vi "SaveGeneralConfigData.vi"(10 "Configurations":T2, 11 "Refnum in":T1) -> (3 "Refnum out":T1)   [LabVIEW 2014]
uses:
  <vilib>/Utility/config.llb/Config Data RefNum.ctl
  <vilib>/Utility/config.llb/Write Key (I32).vi
  <vilib>/Utility/config.llb/NI_LVConfig.lvlib
panel:
  out "error out 3":errorcluster
  out "error out 2":errorcluster
  out "error out":errorcluster
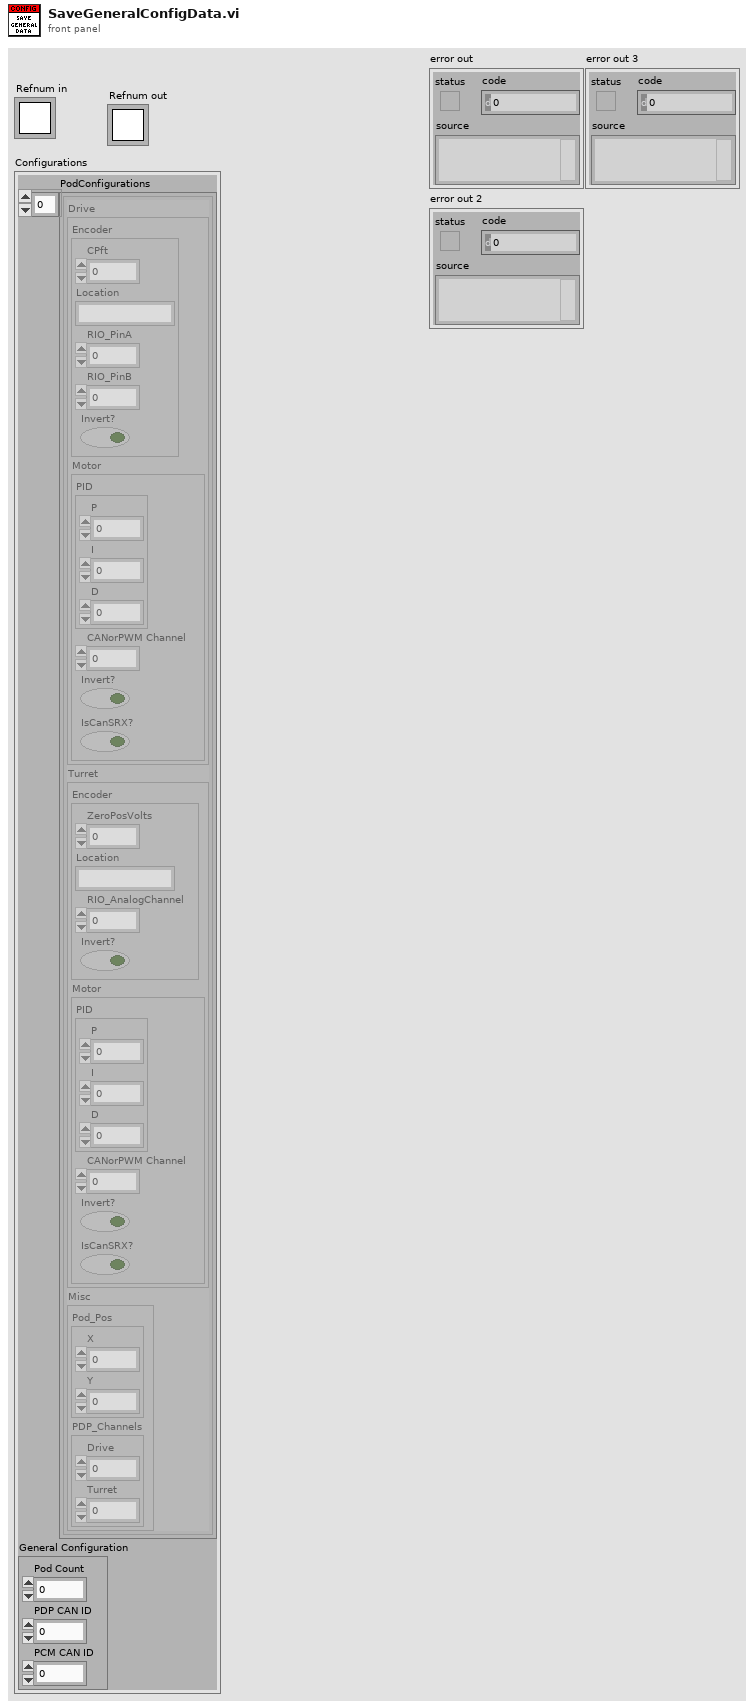
[diagram p1: front panel]
types:
  T1 = typedef "NI_LVConfig.lvlib/Config Data RefNum.ctl" = refnum<k1>
  T2 = cluster{"PodConfigurations":cluster{"Drive":cluster{"Encoder":cluster{"CPft":dbl, "Location":string, "RIO_PinA":i32, "RIO_PinB":i32, "Invert?":bool}, "Motor":cluster{"PID":cluster{"P":dbl, "I":dbl, "D":dbl}, "CANorPWM Channel":i32, "Invert?":bool, "IsCanSRX?":bool}}, "Turret":cluster{"Encoder":cluster{"ZeroPosVolts":dbl, "Location":string, "RIO_AnalogChannel":i32, "Invert?":bool}, "Motor":cluster{"PID":cluster{"P":dbl, "I":dbl, "D":dbl}, "CANorPWM Channel":i32, "Invert?":bool, "IsCanSRX?":bool}}, "Misc":cluster{"Pod_Pos":cluster{"X":dbl, "Y":dbl}, "PDP_Channels":cluster{"Drive":i32, "Turret":i32}}}[], "General Configuration":cluster{"Pod Count":i32, "PDP CAN ID":i32, "PCM CAN ID":i32}}
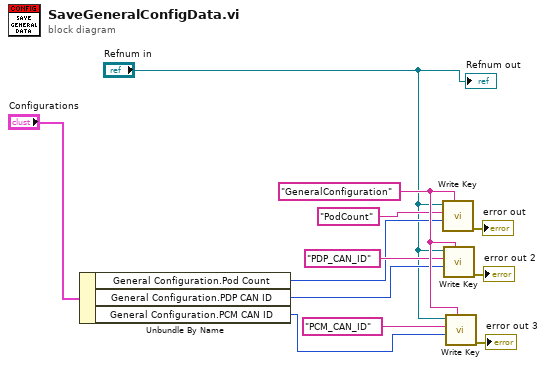
[diagram p0: block diagram]
diagram:
  w12 = "GeneralConfiguration"
  n1 = Unbundle By Name("Configurations") -> ("General Configuration.Pod Count"=w7:i32, "General Configuration.PDP CAN ID"=w9:i32, "General Configuration.PCM CAN ID"=w11:i32)
  n2 = call-poly <vilib>:"Write Key.vi"("section"=w12, "value"=w7, "key"="PodCount", "refnum"="Refnum in") -> ("error out"=→"error out":errorcluster)  [unwired: 5 in, 2 out]
  n3 = call-poly <vilib>:"Write Key.vi"("section"=w12, "value"=w9, "key"="PDP_CAN_ID", "refnum"="Refnum in") -> ("error out"=→"error out 2":errorcluster)  [unwired: 5 in, 2 out]
  n4 = call-poly <vilib>:"Write Key.vi"("section"=w12, "value"=w11, "key"="PCM_CAN_ID", "refnum"="Refnum in") -> ("error out"=→"error out 3":errorcluster)  [unwired: 5 in, 2 out]
  "Refnum out" <- "Refnum in"
